vi "Extract Stage Positions.vi"(11 "Table Stages":T3) -> (1 "Z Stage.Position":dbl, 2 "Y Stage.Position":dbl, 3 "X Stage.Position":dbl)   [LabVIEW 2018]
uses:
  Hardware Mfg/Thorlabs Translation Stages/Controls/Translation Stage Cluster.ctl
  Controls/Translation Stage Types.ctl
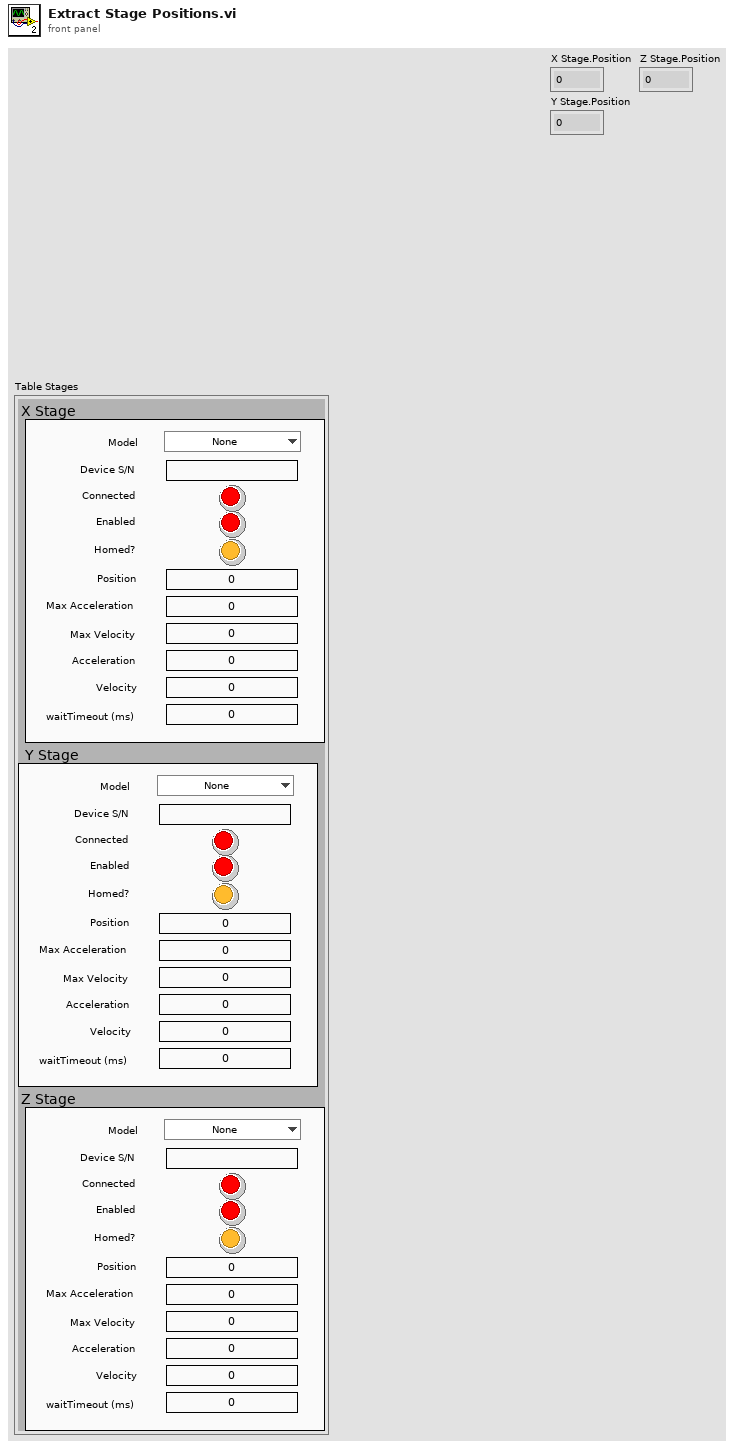
[diagram p1: front panel]
types:
  T1 = typedef "Translation Stage Cluster.ctl" = cluster{"Position":dbl, "Is.Enabled?":bool, "Is.Connected?":bool, "Device SN":string, "AccelerationMaximum":dbl, "VelocityMaximum":dbl, "Acceleration":dbl, "Velocity":dbl, "waitTimeout (ms)":i32, "Model":T2, "Is.Homed?":bool}
  T2 = typedef "Translation Stage Types.ctl" = enum16{"None", "Thorlabs LTS", "Thorlabs MLJ"}
  T3 = cluster{"X Stage":T1, "Y Stage":T1, "Z Stage":T1}
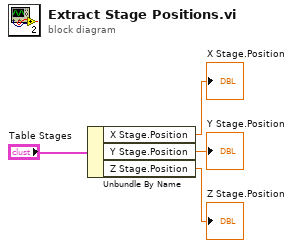
[diagram p0: block diagram]
diagram:
  n1 = Unbundle By Name("Table Stages") -> ("X Stage.Position"=→"X Stage.Position":dbl, "Y Stage.Position"=→"Y Stage.Position":dbl, "Z Stage.Position"=→"Z Stage.Position":dbl)
